vi "GCMPlugin_Run.vi"(8 "error in (no error)":errorcluster, 9 "EventsOut":T1, 11 "_LVCMPlugin in":refnum<class "GCMPlugin.lvclass">) -> (0 "error out":errorcluster, 3 "_LVCMPlugin out":refnum<class "GCMPlugin.lvclass">)   [LabVIEW 2014, in "GCMPlugin.lvclass"]
doc: "Runs the plugin by running the VI provided by GCMPlugin_GetInterfacePath.vi method."
uses:
  GCMPlugin/GCMPlugin.lvclass
  GCMPlugin_EventsOut.ctl
  GCMPlugin/GCMPlugin.lvclass/GCMPlugin.ctl
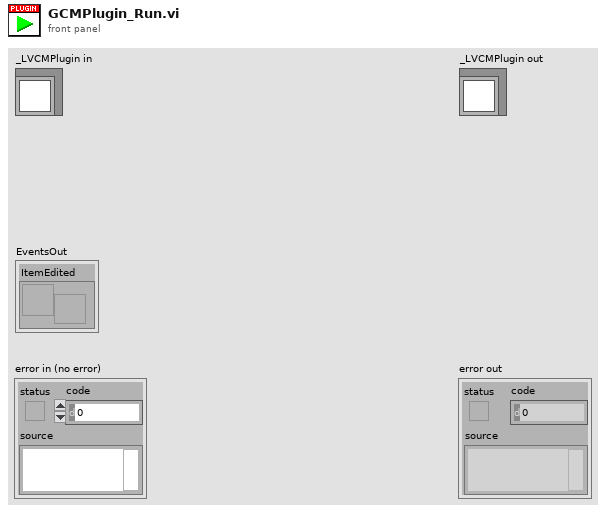
[diagram p1: front panel]
types:
  T1 = typedef "GCMPlugin.lvclass/GCMPlugin_EventsOut.ctl" = cluster{"ItemEdited":refnum<user-event>}
  T2 = typedef "GCMPlugin.lvclass/GCMPlugin_EventsIn.ctl" = cluster{"Stop":refnum<user-event>, "ItemSelected":refnum<user-event>, "ItemDeselected":refnum<user-event>, "PluginActivated":refnum<user-event>, "PluginDeactivated":refnum<user-event>}
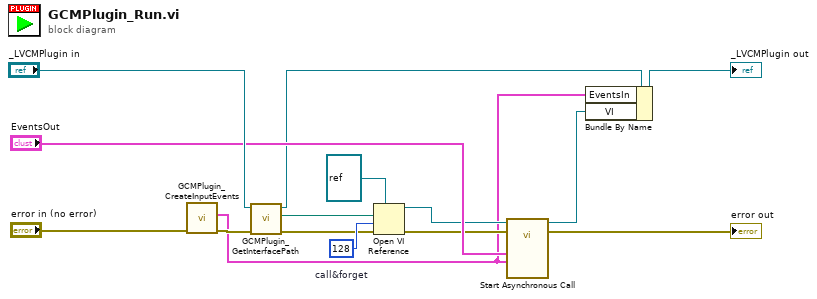
[diagram p0: block diagram]
diagram:
  w10 = 128  # call&forget
  n1 = call "GCMPlugin_CreateInputEvents.vi"("error in (no error)"="error in (no error)") -> ("error out"=w2:errorcluster, "EventsIn"=w1:T2)  [unwired: 9 in]
  n2 = call-dynamic "GCMPlugin_GetInterfacePath.vi"("error in (no error)"=w2, "_LVCMPlugin in"="_LVCMPlugin in") -> ("error out"=w8:errorcluster, "Path"=w7:path, "_LVCMPlugin out"=w4:refnum<class "GCMPlugin.lvclass">)  [unwired: 7 in]
  n3 = Open VI Reference(type specifier VI Refnum (for type only)=refnum<vi> refnum, vi path=w7, options=w10, error in (no error)=w8) -> (vi reference=w5:refnum<vi>, error out=w6:errorcluster)  [unwired: 2 in]
  n4 = call-by-ref "Start Asynchronous Call"(reference=w5, error in=w6, "EventsIn"=w1, "EventsOut"="EventsOut") -> (reference out=w3:refnum<vi>, error out=→"error out":errorcluster)  [unwired: 10 in]
  n5 = Bundle By Name(cluster=w4, "EventsIn"=w1, "VI"=w3) -> (→"_LVCMPlugin out":refnum<class "GCMPlugin.lvclass">)
